vi "Send_ADC.vi"(8 "error in (no error)":errorcluster, 10 "Channel":u8, 11 "Simulated uC in":refnum<class "Simulated uC.lvclass">) -> (0 "error out":errorcluster, 2 "buffer":string, 3 "Simulated uC out":refnum<class "Simulated uC.lvclass">)   [LabVIEW 2019, in "Simulated uC.lvclass"]
uses:
  Simulated uC.lvclass
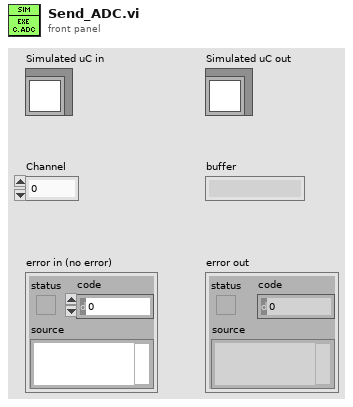
[diagram p1: front panel]
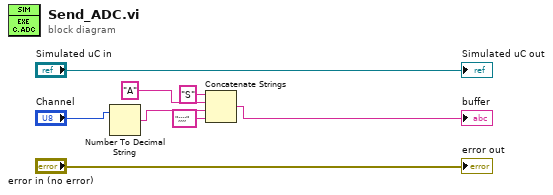
[diagram p0: block diagram]
diagram:
  n1 = Number To Decimal String(number="Channel") -> (decimal integer string=w5:string)  [unwired: 1 in]
  n2 = Concatenate Strings("S" ("string"), "A" ("string"), w5, ";;;;" ("string")) -> (→"buffer":string)
  "error out" <- "error in (no error)"
  "Simulated uC out" <- "Simulated uC in"
